vi "subWindowList.vi"(8 "Error In":errorcluster, 10 "order":T1 items=["CreationOrder", "StackingOrder", "ActivationHistoryOrder"], 11 "QMdiArea In":refnum<class "QMdiArea.lvclass">) -> (0 "Error Out":errorcluster, 2 "Value":refnum<class "QMdiSubWindow.lvclass">[](array[class]), 3 "QMdiArea Out":refnum<class "QMdiArea.lvclass">)   [LabVIEW 2014, in "QMdiArea.lvclass"]
doc: "LabVIEW-specific documentation is not yet available. See <b>https://doc.qt.io/qt-5/qmdiarea.html#subWindowList</b>"
uses:
  QMdiArea.lvclass
  QMdiSubWindow/QMdiSubWindow.lvclass
  WindowOrder.ctl
  LQ Core/LQIdentity/LQIdentity.lvclass/LQIdentity.ctl
  LQ Core/LQ Core.lvlib
  LQ Core/LQIdentity/LQIdentity.lvclass
  LQ Core/LQCoreEngine/LQCoreEngine.lvclass
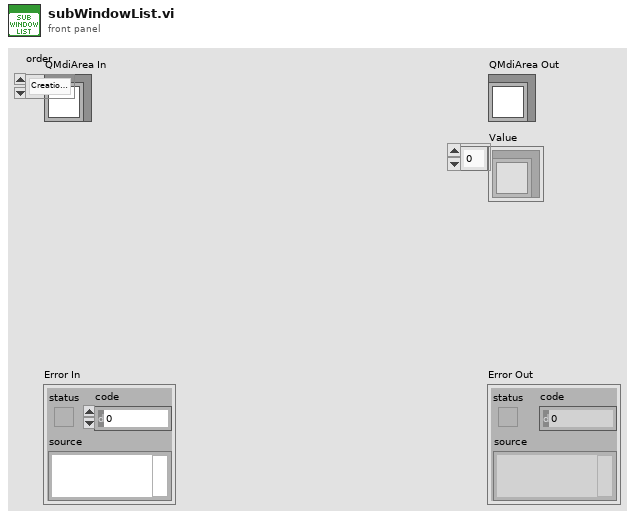
[diagram p1: front panel]
types:
  T1 = typedef "QMdiArea.lvclass/WindowOrder.ctl" = i32
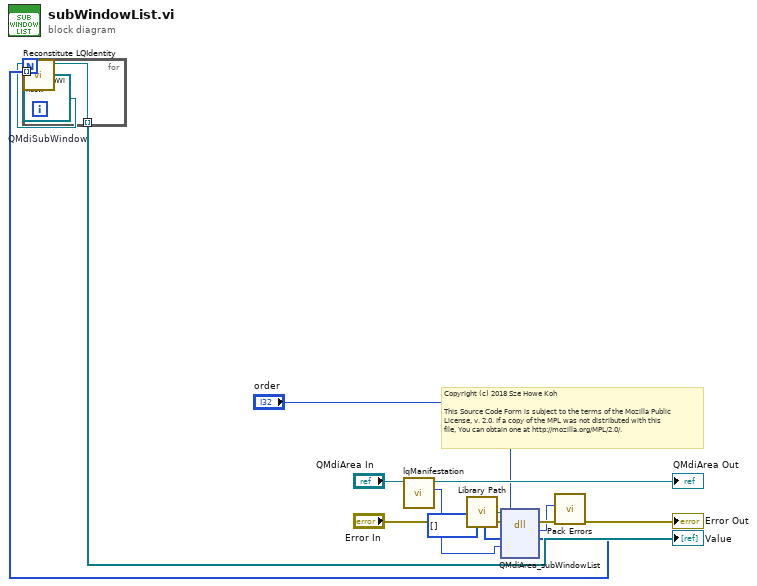
[diagram p0: block diagram]
diagram:
  # "Copyright (c) 2018 Sze Howe Koh\n\nThis Source Code Form is subject to the terms of the Mozilla Public\nLicense, v. 2.0. If a copy of the MPL was not distributed with this\nfile, You can obtain one at http://mozilla.org/MPL/2.0/."
  n1 = call "lqManifestation.vi"("LQIdentity in"="QMdiArea In") -> ("Manifestation"=w8:u64, "LQIdentity out"=→"QMdiArea Out":refnum<class "QMdiArea.lvclass">)  [unwired: 9 in]
  n2 = call "Library Path.vi"() -> ("Library Path"=w9:path)
  n3 = dll-call lib="?" fn="QMdiArea_subWindowList"(path in=w9, error in="Error In", "_retVal"=u64[] [] ("retVal"), "_instance"=w8, "order"="order") -> (error out=w6:errorcluster, w4:i32, "_retVal"=w2:u64[])  [unwired: 3 in, 1 out]
  n4 = for {
    tunnel: [w15] -> w3 mode=indexing
    tunnel: w2 -> [w13] mode=indexing
    w14 = refnum<class "QMdiSubWindow.lvclass"> refnum  # QMdiSubWindow
    n5 = call "Reconstitute LQIdentity.vi"("Manifestation"=w13, "LQIdentity Prototype"=w14) -> ("Reconstituted LQIdentity"=w15:refnum<class "QMdiSubWindow.lvclass">)  [unwired: 8 in, 1 out]
  }
  "Value" <- w3
  n6 = call "Pack Errors.vi"("Error In"=w6, "Error Code"=w4) -> ("Error Out"=→"Error Out":errorcluster)  [unwired: 9 in]
